vi "csmdoc_export_all_csm_VI_description_doc.vi"(5 "LANG ID":string="CＮ") -> ()   [LabVIEW 2017, in "csmdoc.lvlib"]
doc: "Analyze all CSM VIs and export the VI functionality descriptions to a markdown file.\n\n-- <b>Controls</b> --\n- <b>Path</b>: Path to the markdown file describing the functionality of CSM VIs"
uses:
  csmdoc.lvlib
  Communicable State Machine.lvlib
  _Shared/CSM Shared.lvlib
panel:
  in  "Error in":errorcluster caption="error in (no error)"
  out "error out":errorcluster
  out "Array":path[](array[path])
  out "concatenated string":string
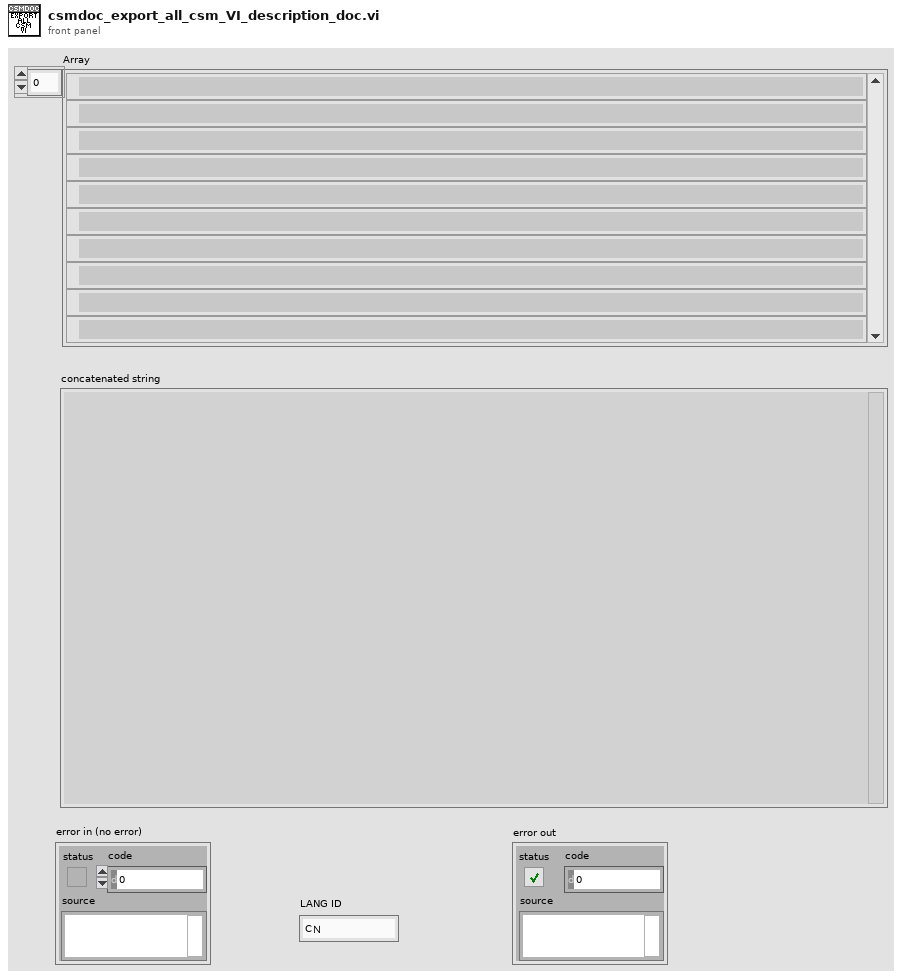
[diagram p1: front panel]
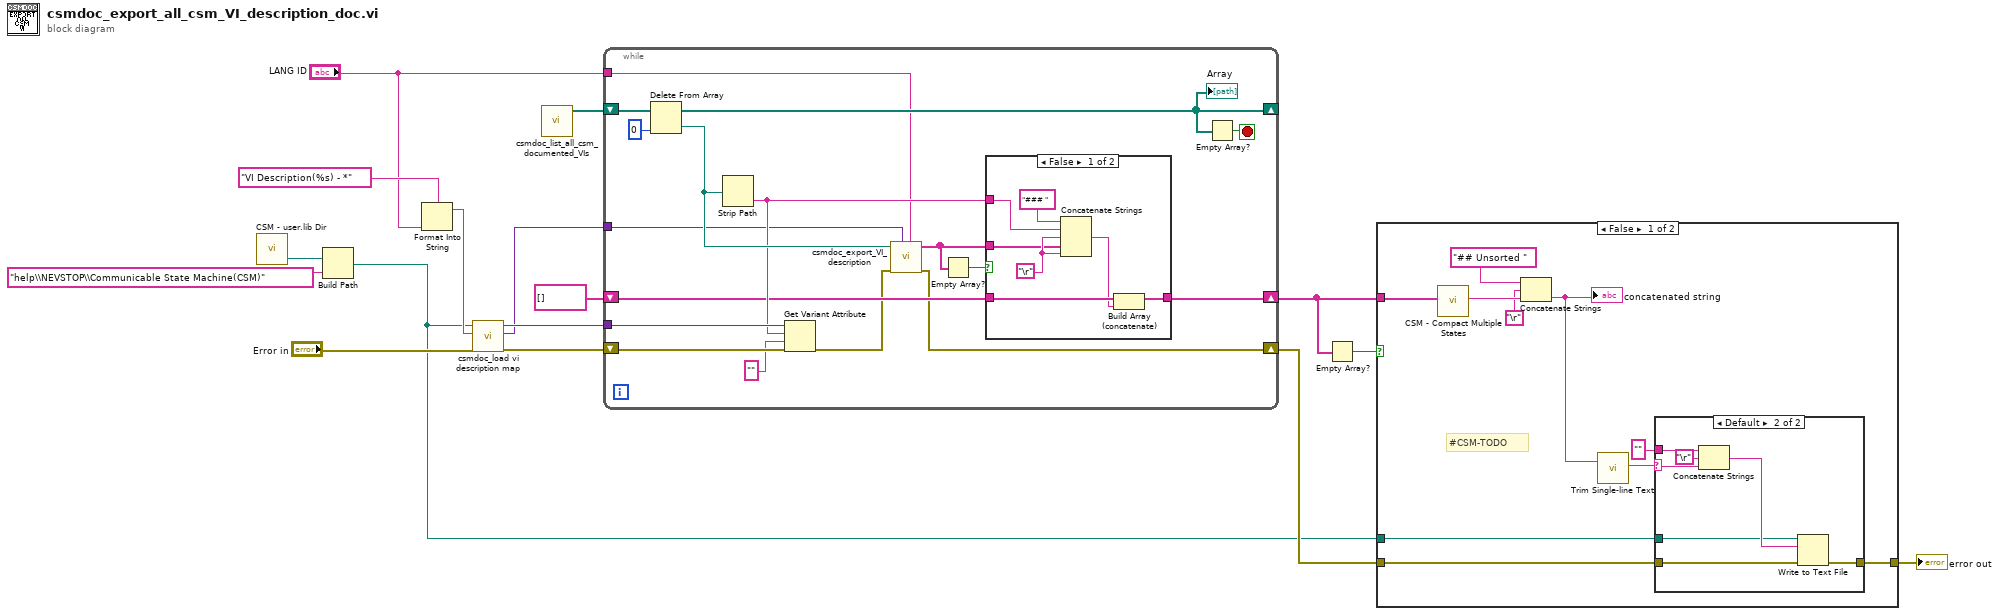
[diagram p0: block diagram]
diagram:
  n1 = call "CSM - user.lib Dir.vi"() -> ("<LabVIEW>"=w5:path)  [unwired: 2 in, 1 out]
  n2 = Build Path(base path=w5, name or relative path="help\\NEVSTOP\\Communicable State Machine(CSM)") -> (appended path=w1:path)
  n3 = Format Into String(format string="VI Description(%s) - *" ("pattern"), "LANG ID") -> (resulting string=w2:string)  [unwired: 2 in, 1 out]
  n4 = call "csmdoc_load vi description map.vi"("Error In"="Error in", "Pattern"=w2, "Path"=w1) -> ("error out"=w13:errorcluster, "NoteMap"=w7:variant, "DescMap"=w15:variant)  [unwired: 6 in]
  n5 = call "csmdoc_list_all_csm_documented_VIs.vi"() -> ("Array"=w16:path[])  [unwired: 11 in]
  n6 = while {
    shift-right: [w30] -> _
    shift-left: w16 -> [w32]
    tunnel: w15 -> [w28]
    shift-right: [w26] -> w9
    shift-left: string[] [] -> [w25]
    shift-right: [w22] -> w12
    shift-left: w13 -> [w24]
    tunnel: w7 -> [w21]
    tunnel: "LANG ID" -> [w17]
    stop <- w31 stop-if-true
    n7 = Delete From Array(array=w32, index=0) -> (deleted portion=w33:path, array with subset deleted=w30:path[])  [unwired: 1 in]
    "Array" <- w30
    n8 = Strip Path(path=w33) -> (name=w27:string)  [unwired: 1 out]
    n9 = Get Variant Attribute(Variant=w28, name=w27, default value (empty Variant)="" ("String"), error in=w24) -> (error out=w23:errorcluster)  [unwired: 3 out]
    n10 = call "csmdoc_export_VI_description.vi"("LANG ID"=w17, "NOTE-Map"=w21, "error in (no error)"=w23, "Path"=w33) -> ("error out"=w22:errorcluster, "Concatenated String"=w20:string[])  [unwired: 6 in]
    n11 = Empty Array?(array=w20) -> (empty?=w19:bool)
    n12 = case shown="False" w19 {
      tunnel: w27 -> [w38 _]
      tunnel: w25 -> [w37 w41]
      tunnel: [w36 w41] -> w26
      tunnel: w20 -> [w34 _]
      frame False {
        w39 = "\r"
        n13 = Concatenate Strings("### " ("string"), w38, w39, w34, w39) -> (w35:string)
        n14 = Build Array (concatenate)(w37, w35) -> (w36:string[])
      }
      frame True {
      }
    }
    n15 = Empty Array?(array=w30) -> (empty?=w31:bool)
  }
  n16 = Empty Array?(array=w9) -> (empty?=w8:bool)
  n17 = case shown="False" w8 {
    tunnel: w1 -> [w47 _]
    tunnel: w12 -> [w46 w60]
    tunnel: [w44 w60] -> w11
    tunnel: w9 -> [w43 _]
    frame False {
      # "#CSM-TODO"
      n18 = call "CSM - Compact Multiple States.vi"("Multiple States"=w43) -> ("States"=w50:string)  [unwired: 9 in]
      n19 = Concatenate Strings("## Unsorted " ("string"), "\r" ("Carriage Return Constant"), w50) -> (w45:string)
      "concatenated string" <- w45
      n20 = call "Trim Single-line Text.vi"("single-line text"=w45) -> ("trimed text"=w48:string)  [unwired: 2 in]
      n21 = case shown="Default" w48 {
        selector: w48 -> [_ w58]
        tunnel: "" ("text") -> [_ w57]
        tunnel: w47 -> [_ w55]
        tunnel: w46 -> [w52 w54]
        tunnel: [w52 w53] -> w44
        frame "" {
        }
        frame Default {
          n22 = Concatenate Strings(w57, "\r", w58) -> (w56:string)
          n23 = Write to Text File(file (use dialog)=w55, text=w56, error in=w54) -> (error out=w53:errorcluster)  [unwired: 1 in, 2 out]
        }
      }
    }
    frame True {
    }
  }
  "error out" <- w11
